vi "CallButton TCP Server.vi"(8 "error in (no error)":errorcluster, 10 "queue in":refnum<queue>, 11 "Boolean in":refnum<vi>) -> (0 "error out":errorcluster)   [LabVIEW 2018]
uses:
  Button Class/TCP Message Payload.ctl
  Button Class/TCP Multiple Connections State.ctl
  Button Class/TCP Multiple Connections Data.ctl
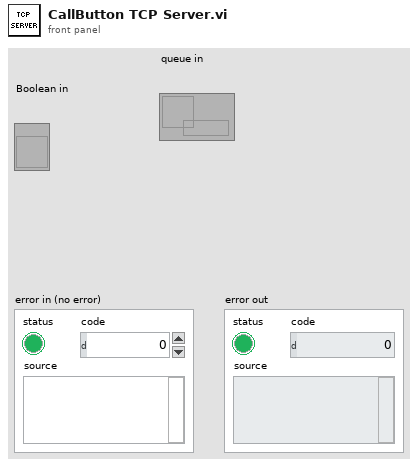
[diagram p1: front panel]
types:
  T1 = typedef "TCP Multiple Connections Data.ctl" = cluster{"Clients":refnum<k5>[], "Listener":refnum<k5>}
  T2 = typedef "TCP Multiple Connections State.ctl" = enum16{"Initialize", "Status Check", "Read Data", "Stop"}
  T3 = typedef "TCP Message Payload.ctl" = cluster{"ID":string, "First Active":timestamp, "Button State":bool}
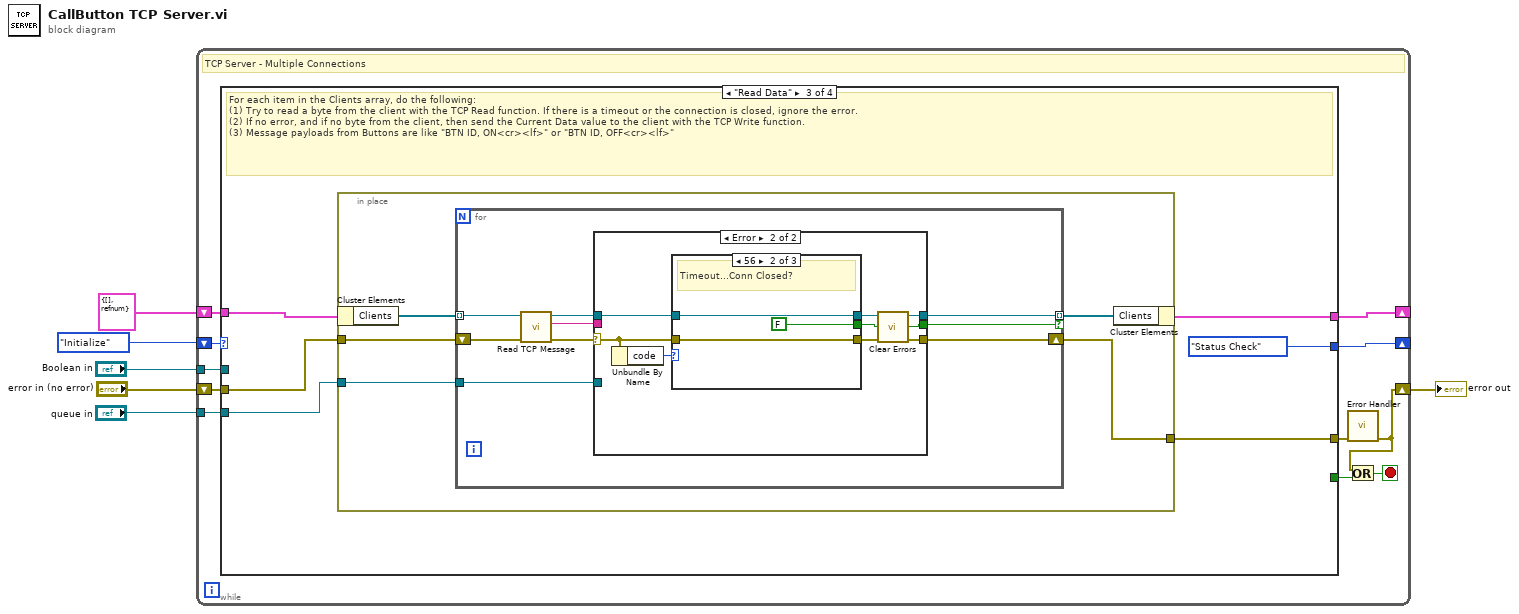
[diagram p0: block diagram]
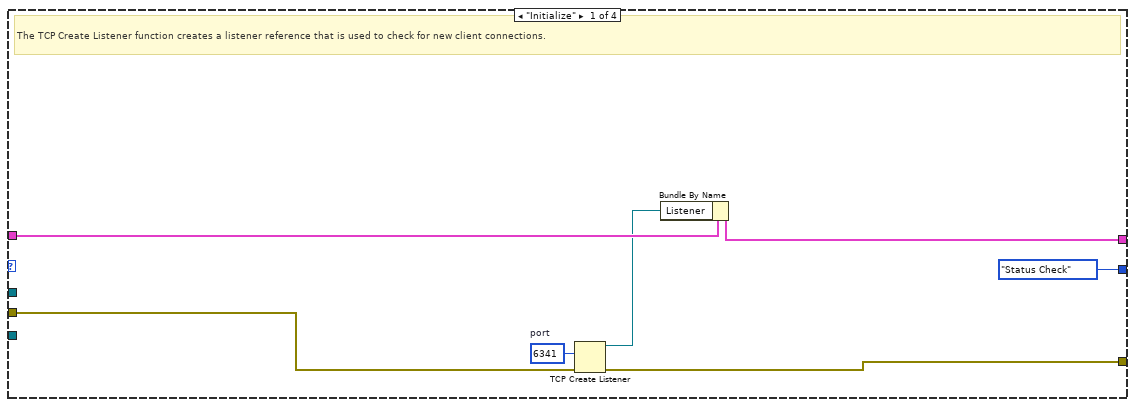
[diagram p2: hidden frame]
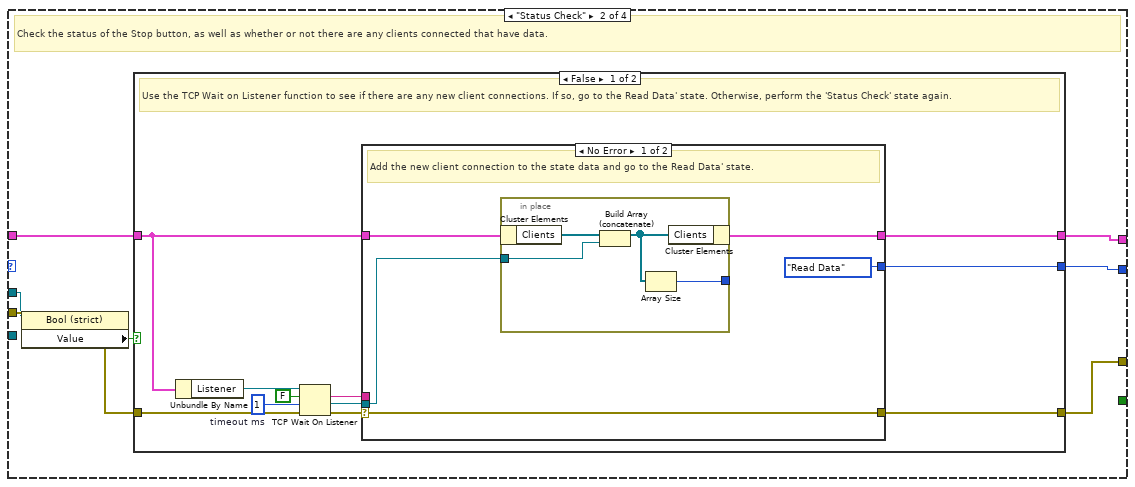
[diagram p3: hidden frame]
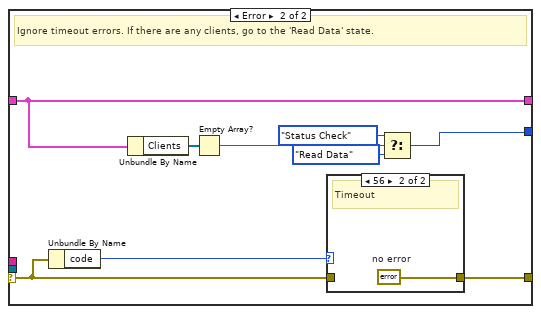
[diagram p4: hidden frame]
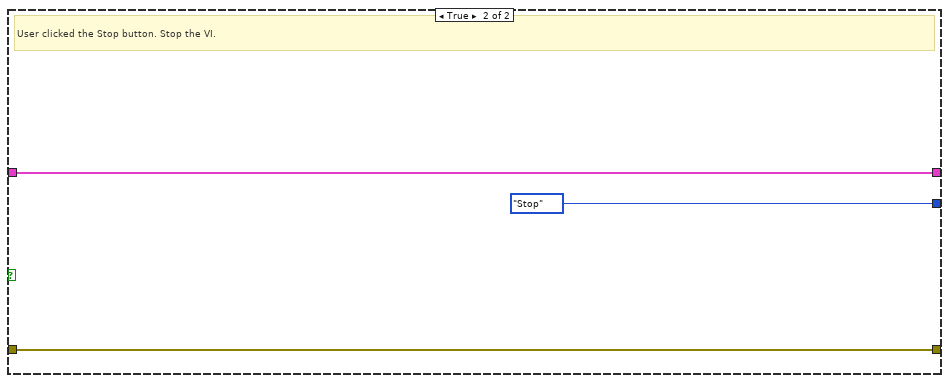
[diagram p6: hidden frame]
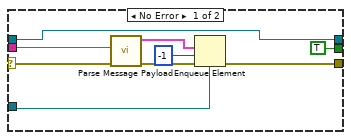
[diagram p7: hidden frame]
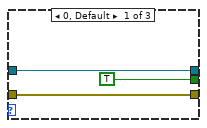
[diagram p8: hidden frame]
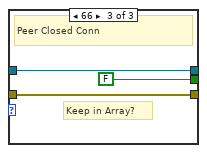
[diagram p9: hidden frame]
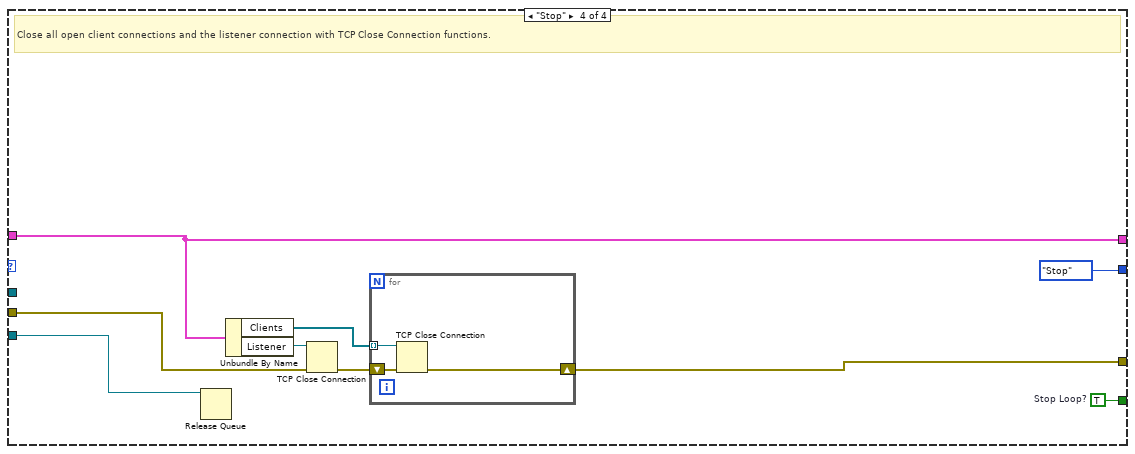
[diagram p10: hidden frame]
diagram:
  n1 = while {
    shift-right: [w11] -> _
    shift-left: TCP_Multiple_Connections_State."Initialize" ("States") -> [w17]
    shift-right: [w15] -> _
    shift-left: T1 {"Clients"=[], "Listener"=refnum} ("Data") -> [w16]
    shift-right: [w7] -> w5
    shift-left: "error in (no error)" -> [w14]
    tunnel: "queue in" -> [w10]
    tunnel: "Boolean in" -> [w9]
    stop <- w12 stop-if-true
    # "TCP Server - Multiple Connections"
    n2 = case shown="\"Read Data\"" w17 {
      tunnel: [TCP_Multiple_Connections_State."Status Check" ("States") w31 TCP_Multiple_Connections_State."Status Check" ("States") TCP_Multiple_Connections_State."Stop" ("(Value Not Used)")] -> w11
      tunnel: [_ _ _ w119] -> w13
      tunnel: w16 -> [w22 w28 w69 w118]
      tunnel: [w21 w27 w68 w118] -> w15
      tunnel: w14 -> [w24 w30 w71 w117]
      tunnel: [w23 w29 w70 w115] -> w8
      tunnel: w10 -> [_ _ w66 w111]
      tunnel: w9 -> [_ w25 _ _]
      frame "Initialize" {
        w19 = u16 6341  # port
        # "The TCP Create Listener function creates a listener reference that is used to check for new client connections."
        n3 = TCP Create Listener(8:w24, 10:w19) -> (0:w23:errorcluster, 3:w20:refnum<k5>)  [unwired: 4 out]
        n4 = Bundle By Name(cluster=w22, "Listener"=w20) -> (w21:T1)
      }
      frame "Status Check" {
        # "Check the status of the Stop button, as well as whether or not there are any clients connected that have data."
        n5 = property on="Property Node" class="Bool (strict)"(reference=w25) -> ("Value"=w26:bool)  [unwired: 1 in, 2 out]
        n6 = case shown="False" w26 {
          tunnel: [w42 TCP_Multiple_Connections_State."Stop" ("States")] -> w31
          tunnel: w30 -> [w41 w65]
          tunnel: [w34 w65] -> w29
          tunnel: w28 -> [w37 w64]
          tunnel: [w36 w64] -> w27
          frame False {
            w40 = 1  # timeout ms
            # "Use the TCP Wait on Listener function to see if there are any new client connections. If so, go to the Read Data' state. Otherwise, perform the 'Status Check' state again."
            n7 = Unbundle By Name(w37) -> ("Listener"=w35:refnum<k5>)
            n8 = TCP Wait On Listener(8:w41, 9:w40, 10:FALSE ("resolve remote address (T)"), 11:w35) -> (0:w39:errorcluster, 2:w33:string, 4:w38:refnum<k5>)  [unwired: 2 out]
            n9 = case shown="No Error" w39 {
              selector: w39 -> [w45 w60]
              tunnel: [TCP_Multiple_Connections_State."Read Data" ("Initial State") w54] -> w42
              tunnel: w38 -> [w46 _]
              tunnel: w37 -> [w47 w57]
              tunnel: [w44 w57] -> w36
              tunnel: [w45 w58] -> w34
              tunnel: w33 -> [_ _]
              frame No Error {
                # "Add the new client connection to the state data and go to the Read Data' state."
                n10 = in-place {
                  in-place-border: w46 -> [w50]
                  in-place-border: [w48] -> _
                  n11 = in-place-cluster #1(w47) -> ("Clients"=w51:refnum<k5>[])
                  n12 = Build Array (concatenate)(w51, w50) -> (w49:refnum<k5>[])
                  n13 = Array Size(array=w49) -> (size(s)=w48:i32)
                  n14 = in-place-cluster #1("Clients"=w49) -> (w44:T1)
                }
              }
              frame Error {
                # "Ignore timeout errors. If there are any clients, go to the 'Read Data' state."
                n15 = Unbundle By Name(w60) -> ("code"=w59:i32)
                n16 = Unbundle By Name(w57) -> ("Clients"=w56:refnum<k5>[])
                n17 = Empty Array?(array=w56) -> (empty?=w55:bool)
                n18 = case shown="56" w59 {
                  tunnel: w60 -> [w61 _]
                  tunnel: [w61 w62] -> w58
                  frame Default {
                  }
                  frame 56 {
                    w62 = errorcluster {"status"=FALSE, "code"=0, "source"=""}  # no error
                    # "Timeout"
                  }
                }
                n19 = Select(t=TCP_Multiple_Connections_State."Status Check" ("States"), s=w55, f=TCP_Multiple_Connections_State."Read Data" ("Initial State")) -> (s? t:f=w54:T2)
              }
            }
          }
          frame True {
            # "User clicked the Stop button. Stop the VI."
          }
        }
      }
      frame "Read Data" {
        # "For each item in the Clients array, do the following:\n(1) Try to read a byte from the client with the TCP Read function. If there is a timeout or the connection is closed, ignore the error. \n(2) If no error, and if no byte from the client, then send the Current Data value to the client with the TCP Write function.\n(3) Message payloads from Buttons are like \"BTN ID, ON<cr><lf>\" or \"BTN ID, OFF<cr><lf>\""
        n20 = in-place {
          in-place-border: w71 -> [w76]
          in-place-border: [w75] -> w70
          in-place-border: w66 -> [w72]
          n21 = in-place-cluster #2(w69) -> ("Clients"=w74:refnum<k5>[])
          n22 = for {
            tunnel: w74 -> [w85] mode=indexing
            shift-right: [w80] -> w75
            shift-left: w76 -> [w84]
            tunnel: [w79] -> w73 mode=indexing if=w77
            tunnel: w72 -> [w81]
            n23 = call "Read TCP Message.vi"("error in (no error)"=w84, "TCP Network Connection in"=w85) -> ("error out"=w82:errorcluster, "data out"=w78:string, "connection ID out"=w83:refnum<k5>)  [unwired: 7 in]
            n24 = case shown="Error" w82 {
              selector: w82 -> [w94 w97]
              tunnel: [w89 w98] -> w80
              tunnel: w83 -> [w87 w100]
              tunnel: w78 -> [w93 _]
              tunnel: [w87 w99] -> w79
              tunnel: w81 -> [w92 _]
              tunnel: [TRUE w95] -> w77
              frame No Error {
                n25 = call "Parse Message Payload.vi"("error in"=w94, "TCP Message In"=w93) -> ("error out"=w90:errorcluster, "Parsed Message"=w88:T3)  [unwired: 8 in]
                n26 = Enqueue Element(queue=w92, element=w88, timeout in ms (-1)=-1, error in (no error)=w90) -> (error out=w89:errorcluster)  [unwired: 2 out]
              }
              frame Error {
                n27 = Unbundle By Name(w97) -> ("code"=w101:i32)
                n28 = case shown="56" w101 {
                  tunnel: w100 -> [w103 w107 w109]
                  tunnel: [w103 w107 w109] -> w99
                  tunnel: w97 -> [w104 w106 w110]
                  tunnel: [w104 w106 w110] -> w96
                  tunnel: [TRUE FALSE FALSE] -> w95
                  frame 0, Default {
                  }
                  frame 56 {
                    # "Timeout...Conn Closed?"
                  }
                  frame 66 {
                    # "Keep in Array?"
                    # "Peer Closed Conn"
                  }
                }
                n29 = call <vilib>:"Clear Errors.vi"("error in (no error)"=w96) -> ("error out"=w98:errorcluster)  [unwired: 5 in, 1 out]
              }
            }
          }
          n30 = in-place-cluster #2("Clients"=w73) -> (w68:T1)
        }
      }
      frame "Stop" {
        w119 = TRUE  # Stop Loop?
        # "Close all open client connections and the listener connection with TCP Close Connection functions."
        n31 = Release Queue(queue=w111) -> ()  [unwired: 2 in, 3 out]
        n32 = Unbundle By Name(w118) -> ("Clients"=w116:refnum<k5>[], "Listener"=w113:refnum<k5>)
        n33 = TCP Close Connection(connection ID=w113, error in (no error)=w117) -> (error out=w114:errorcluster)  [unwired: 1 in, 1 out]
        n34 = for {
          shift-right: [w121] -> w115
          shift-left: w114 -> [w122]
          tunnel: w116 -> [w120] mode=indexing
          n35 = TCP Close Connection(connection ID=w120, error in (no error)=w122) -> (error out=w121:errorcluster)  [unwired: 1 in, 1 out]
        }
      }
    }
    n36 = call "Error Handler.vi"("error in (no error)"=w8) -> ("error out (no error)"=w7:errorcluster)  [unwired: 10 in]
    n37 = Or(x=w7, y=w13) -> (x .or. y?=w12:bool)
  }
  "error out" <- w5
